vi "Simple on-off.vi"() -> ()   [LabVIEW 2021]
panel:
  out "s? t:f":string
  out "Boolean 2":bool
  out "return count":u32
  in  "Boolean":bool
  in  "stop":bool
  in  "VISA resource name":refnum<visa-resource-name>
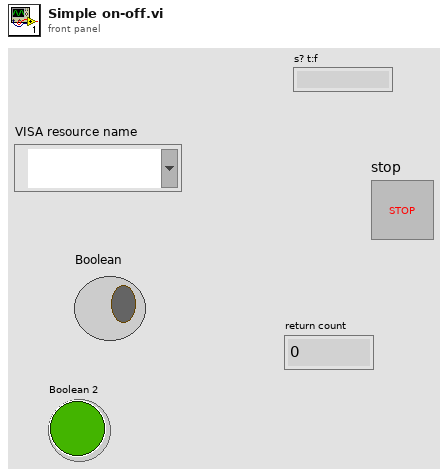
[diagram p1: front panel]
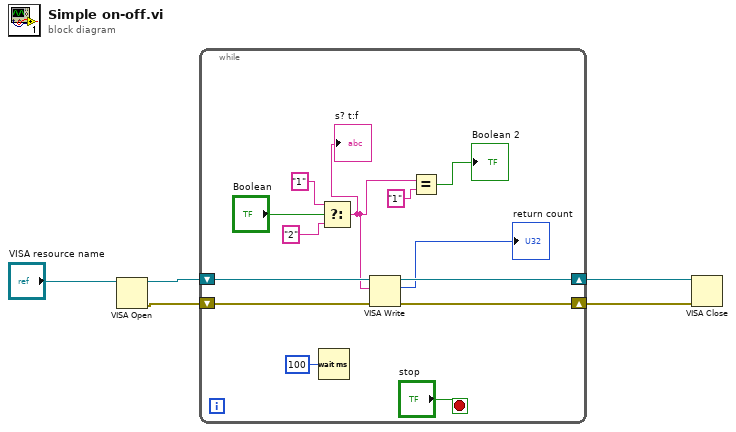
[diagram p0: block diagram]
diagram:
  n1 = VISA Open(VISA resource name="VISA resource name") -> (VISA resource name=w5:refnum<visa-resource-name>, error out=w2:errorcluster)  [unwired: 4 in]
  n2 = while {
    shift-right: [w17] -> w4
    shift-left: w5 -> [w18]
    shift-right: [w16] -> w3
    shift-left: w2 -> [w15]
    stop <- "stop" stop-if-true
    n3 = Wait (ms)(milliseconds to wait=u32 100) -> ()  [unwired: 1 out]
    n4 = Select(t="1", s="Boolean", f="2") -> (s? t:f=w8:string)
    "s? t:f" <- w8
    n5 = VISA Write(VISA resource name=w18, write buffer=w8, error in (no error)=w15) -> (VISA resource name out=w17:refnum<visa-resource-name>, return count=→"return count":u32, error out=w16:errorcluster)
    n6 = Equal?(x=w8, y="1") -> (x = y?=→"Boolean 2":bool)
  }
  n7 = VISA Close(VISA resource name=w4, error in (no error)=w3) -> ()  [unwired: 1 out]
